vi "Read Control Label.vi"(8 "error in (no error)":errorcluster, 11 "ControlDragSourceUpdateMsg In":refnum<class "ControlDragSourceUpdateMsg.lvclass">) -> (0 "error out":errorcluster, 2 "Control Label":string, 3 "ControlDragSourceUpdateMsg Out":refnum<class "ControlDragSourceUpdateMsg.lvclass">)   [LabVIEW 2020, in "MVA Framework.lvlib" / "ActorEvents.lvlib" / "ControlDragSourceUpdateMsg.lvclass"]
uses:
  ControlDragSourceUpdateMsg.lvclass
  ControlDragSourceUpdateMsg.lvclass/ControlDragSourceUpdateMsg.ctl
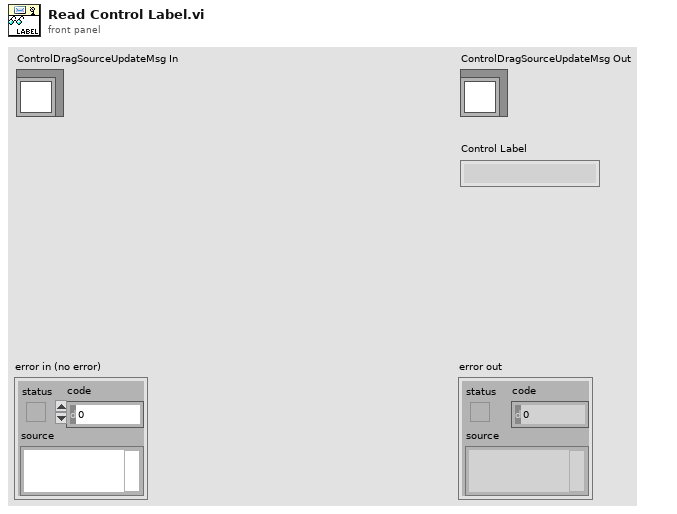
[diagram p1: front panel]
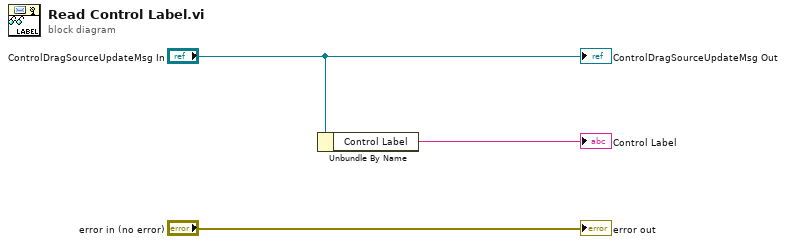
[diagram p0: block diagram]
diagram:
  n1 = Unbundle By Name("ControlDragSourceUpdateMsg In") -> ("Control Label"=→"Control Label":string)
  "error out" <- "error in (no error)"
  "ControlDragSourceUpdateMsg Out" <- "ControlDragSourceUpdateMsg In"
